vi "Controller - Launch Distributor (ROOT).vi"(8 "error in":errorcluster) -> (0 "error out":errorcluster)   [LabVIEW 2023, in "Controller.lvlib" / "Controller.lvclass"]
uses:
  Controller.lvclass
  Message_Distributor/Message_Distributor_Class.lvclass
  C:/Program Files/National Instruments/LabVIEW 2023/vi.lib/ActorFramework/Actor/Actor.lvclass
  Controller - Ctrl - FGV - Action.ctl
  Message_Distributor/Message_Distributor_Class.lvclass/Message_Distributor_Class.ctl
  <vilib>/Utility/error.llb/Trim Whitespace.vi
  <vilib>/Utility/error.llb/Trim Whitespace One-Sided.vi
  <vilib>/Utility/LVClass/Get LV Class Name.vi
  <vilib>/ActorFramework/Actor/Actor.lvclass
panel:
  # "LAUNCHER"
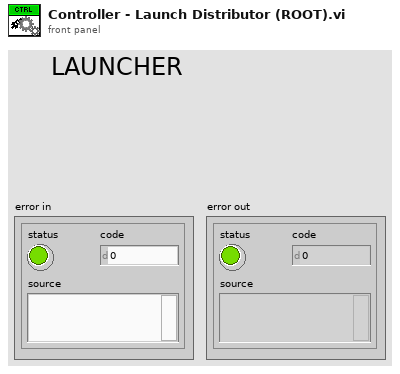
[diagram p1: front panel]
types:
  T1 = typedef "Controller.lvlib/Controller.lvclass/Controller - Ctrl - FGV - Action.ctl" = enum16{"Int", "Get"}
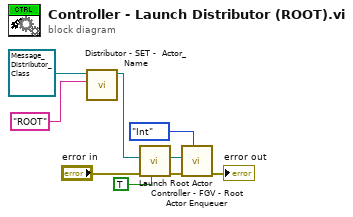
[diagram p0: block diagram]
diagram:
  n1 = call "Distributor - SET -  Actor_Name.vi"("Actor_Name"="ROOT", "Parent_Class in"=refnum<class "Message_Distributor_Class.lvclass"> refnum ("Actor_Parent.lvlib:Parent_Class.lvclass")) -> ("Parent_Class out"=w2:refnum<class "Message_Distributor_Class.lvclass">)  [unwired: 8 in, 1 out]
  n2 = call <vilib>:"Launch Root Actor.vi"("Open Actor Core front panel? (F)"=TRUE, "error in (no error)"="error in", "Actor"=w2) -> ("error out"=w8:errorcluster, "Actor's Enqueuer"=w7:refnum<class "Message Enqueuer.lvclass">)  [unwired: 7 in]
  n3 = call "Controller - FGV - Root Actor Enqueuer.vi"("Action"=Controller_-_Ctrl_-_FGV_-_Action."Int", "error in"=w8, "Actor's Enqueuer"=w7) -> ("error out"=→"error out":errorcluster)  [unwired: 7 in, 1 out]
